vi "formatAccelerometer.vi"(2 "error in (no error)":errorcluster, 3 "SPIDevRef":T1) -> (0 "error out":errorcluster, 1 "SPIDevRef out":T1)   [LabVIEW 2012]
uses:
  <vilib>/Rock Robotics/WPI/SPI/WPI_SPIDevRef.ctl
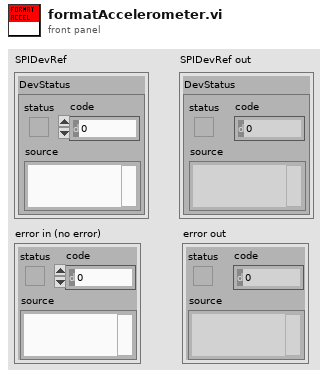
[diagram p1: front panel]
types:
  T1 = typedef "WPI_SPIDevRef.ctl" = cluster{"DevStatus":errorcluster}
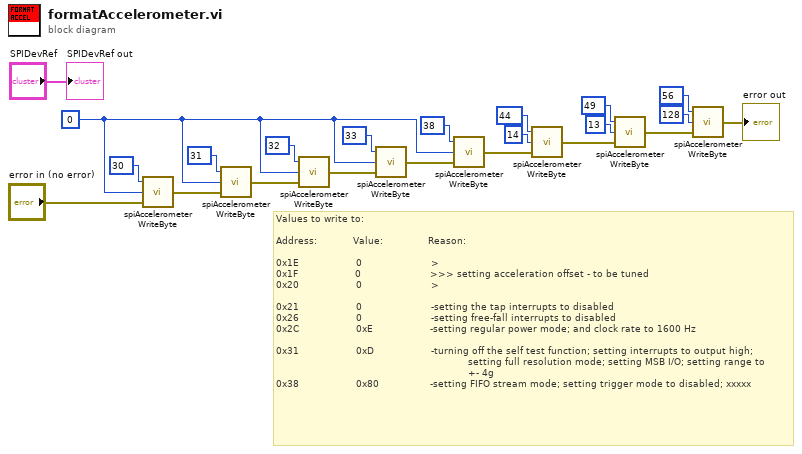
[diagram p0: block diagram]
diagram:
  w2 = u16 0 ("Data")
  # "Values to write to:\n\nAddress:            Value:               Reason:\n\n0x1E                   0                       >\n0x1F                   0                       >>> setting acceleration offset - to be tuned\n0x20                   0                       >\n\n0x21                   0                       -setting the tap interrupts to disabled\n0x26                   0                       -setting free-fall interrupts to disabled\n0x2C                   0xE                   -setting regular power mode; and clock rate to 1600 Hz \n\n0x31                   0xD                   -turning off the self test function; setting interrupts to output high;\n                                                                setting full resolution mode; setting MSB I/O; setting range to\n                                                                +- 4g\n0x38                   0x80                 -setting FIFO stream mode; setting trigger mode to disabled; xxxxx"
  n1 = call "spiAccelerometerWriteByte.vi"("error in (no error)"="error in (no error)", "Data"=w2, "Address"=u16 30) -> ("error out"=w18:errorcluster)
  n2 = call "spiAccelerometerWriteByte.vi"("error in (no error)"=w18, "Data"=w2, "Address"=u16 31) -> ("error out"=w16:errorcluster)
  n3 = call "spiAccelerometerWriteByte.vi"("error in (no error)"=w16, "Data"=w2, "Address"=u16 32) -> ("error out"=w9:errorcluster)
  n4 = call "spiAccelerometerWriteByte.vi"("error in (no error)"=w9, "Data"=w2, "Address"=u16 33) -> ("error out"=w13:errorcluster)
  n5 = call "spiAccelerometerWriteByte.vi"("error in (no error)"=w13, "Data"=w2, "Address"=u16 38) -> ("error out"=w10:errorcluster)
  n6 = call "spiAccelerometerWriteByte.vi"("error in (no error)"=w10, "Data"=u16 14, "Address"=u16 44) -> ("error out"=w3:errorcluster)
  n7 = call "spiAccelerometerWriteByte.vi"("error in (no error)"=w3, "Data"=u16 13, "Address"=u16 49) -> ("error out"=w4:errorcluster)
  n8 = call "spiAccelerometerWriteByte.vi"("error in (no error)"=w4, "Data"=u16 128, "Address"=u16 56) -> ("error out"=→"error out":errorcluster)
  "SPIDevRef out" <- "SPIDevRef"
